vi "non_FPGA_VI.vi"() -> ()   [LabVIEW 2020]
uses:
  <vilib>/Analysis/NI_AALBase.lvlib
panel:
  out "sorted array":sgl[](graph)
  out "sorted array index":i32[](array[numeric])
  out "sorted array real":sgl[](array[numeric])
  out "sorted array":dbl[](array[numeric])
  out "uniform white noise":dbl[](array[numeric])
  out "array input":dbl[](graph)
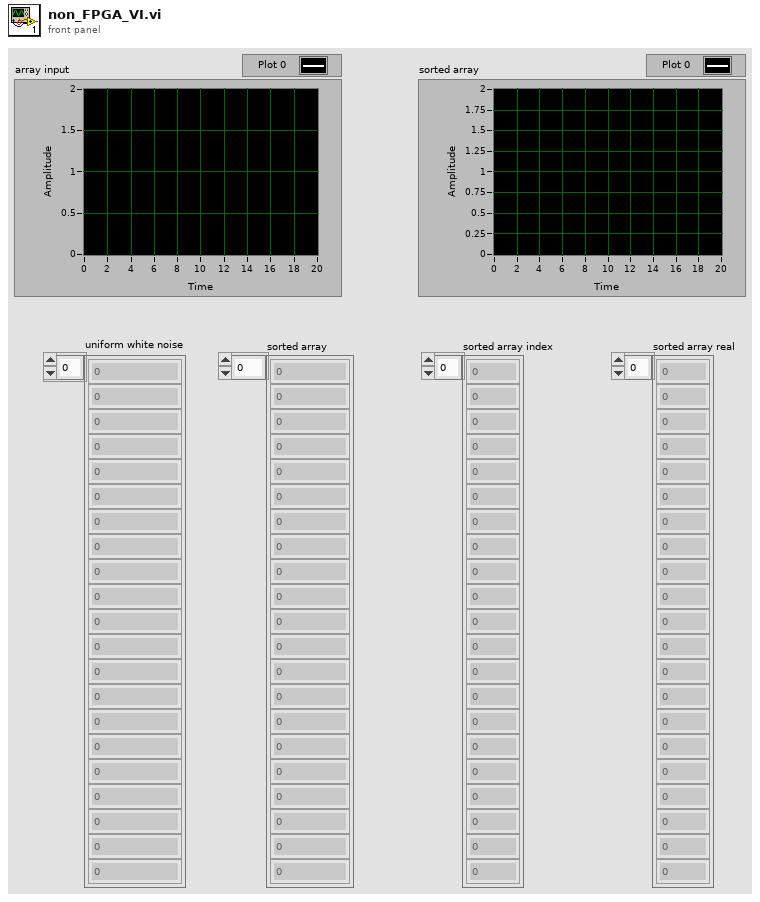
[diagram p1: front panel]
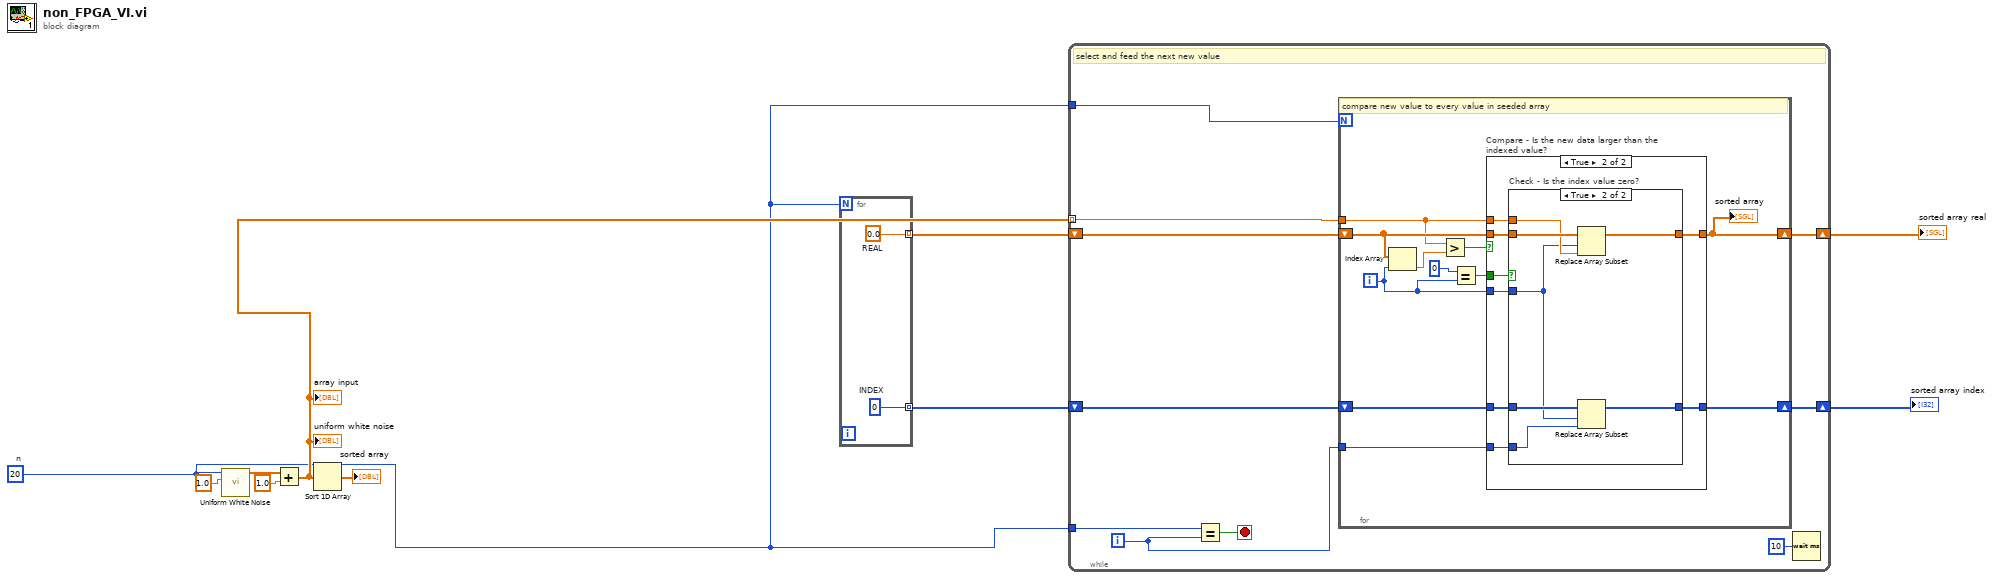
[diagram p0: block diagram]
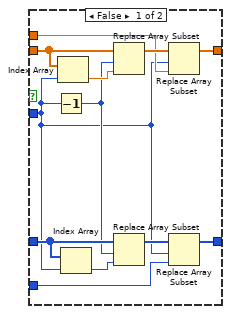
[diagram p3: hidden frame]
diagram:
  w1 = 20  # n
  n1 = call <vilib>:"Uniform White Noise.vi"("amplitude"=1.0, "samples"=w1) -> ("uniform white noise"=w7:dbl[])  [unwired: 8 in, 1 out]
  n2 = Add(x=w7, y=1.0 ("amplitude")) -> (x+y=w3:dbl[])
  "array input" <- w3
  "uniform white noise" <- w3
  n3 = Sort 1D Array(array=w3) -> (sorted array=→"sorted array":dbl[])
  n4 = for {
    N: w1 -> [_]
    tunnel: [w12] -> w5 mode=indexing
    tunnel: [w11] -> w6 mode=indexing
    w11 = 0  # INDEX
    w12 = sgl 0.0  # REAL
  }
  n5 = while {
    shift-right: [w15] -> w2
    shift-left: w5 -> [w22]
    shift-right: [w21] -> w4
    shift-left: w6 -> [w20]
    tunnel: w1 -> [w18]
    tunnel: w3 -> [w13] mode=indexing
    tunnel: w1 -> [w16]
    i -> [w19]
    stop <- w17 stop-if-true
    # "select and feed the next new value"
    n6 = Equal?(x=w18, y=w19) -> (x = y?=w17:bool)
    n7 = for {
      N: w16 -> [_]
      tunnel: w13 -> [w30]
      shift-right: [w29] -> w15
      shift-left: w22 -> [w31]
      tunnel: w19 -> [w27]
      shift-right: [w25] -> w21
      shift-left: w20 -> [w26]
      i -> [w28]
      # "compare new value to every value in seeded array"
      n8 = Index Array(array=w31, index=w28) -> (element=w33:sgl)
      n9 = Greater?(x=w30, y=w33) -> (0:w32:bool)
      n10 = Equal?(x=0, y=w28) -> (x = y?=w23:bool)
      n11 = case "Compare - Is the new data larger than the indexed value?" shown="True" w32 {
        tunnel: w31 -> [w35 w42]
        tunnel: w23 -> [_ w43]
        tunnel: w30 -> [_ w41]
        tunnel: w28 -> [_ w40]
        tunnel: [w35 w39] -> w29
        tunnel: w27 -> [_ w38]
        tunnel: w26 -> [w34 w37]
        tunnel: [w34 w36] -> w25
        frame False {
        }
        frame True {
          n12 = case "Check - Is the index value zero?" shown="True" w43 {
            tunnel: w42 -> [w55 w62]
            tunnel: w41 -> [w52 w61]
            tunnel: w40 -> [w44 w56]
            tunnel: [w51 w60] -> w39
            tunnel: w38 -> [w46 w59]
            tunnel: w37 -> [w48 w58]
            tunnel: [w47 w57] -> w36
            frame False {
              n13 = Decrement(x=w44) -> (x-1=w45:i32)
              n14 = Index Array(array=w55, index=w44) -> (element=w54:sgl)
              n15 = Index Array(array=w48, index=w44) -> (element=w50:i32)
              n16 = Replace Array Subset(array=w55, new element=w54, index=w45) -> (w53:sgl[])
              n17 = Replace Array Subset(array=w48, new element=w50, index=w45) -> (w49:i32[])
              n18 = Replace Array Subset(array=w53, new element=w52, index=w44) -> (w51:sgl[])
              n19 = Replace Array Subset(array=w49, new element=w46, index=w44) -> (w47:i32[])
            }
            frame True {
              n20 = Replace Array Subset(array=w62, new element=w61, index=w56) -> (w60:sgl[])
              n21 = Replace Array Subset(array=w58, new element=w59, index=w56) -> (w57:i32[])
            }
          }
        }
      }
      "sorted array" <- w29
    }
    n22 = Wait (ms)(milliseconds to wait=u32 10) -> ()  [unwired: 1 out]
  }
  "sorted array real" <- w2
  "sorted array index" <- w4
